vi "UTIL_Test_LUT.vi"() -> ()   [LabVIEW 2024]
uses:
  Control Definitions/Def FullCfg.ctl
  Control Definitions/Def BenchCfg.ctl
  Control Definitions/Def PumpCtlRefs.ctl
  Control Definitions/Def Bench Status.ctl
  Control Definitions/Ded Spec RNG.ctl
  Control Definitions/Ded LUT_Status.ctl
panel:
  out "Spec RNG":T1={"Specs"=[6.885, 6.785, 6.435, 304.0, 296.0], "Index(n)"=2, "LUT Status"={"ChA/!ChB"=FALSE, "Drain/!Fill"=FALSE, "In Range?"=TRUE, "Switch Range?"=FALSE, "Measure R?"=FALSE, "Vaild R?"=FALSE}, "Index(n-1)"=1}
  in  "Level IN inches":dbl=5.0
  in  "ChA/!ChB":bool
  in  "Drain!Fill":bool
  in  "Full Cfg":T3={"Bench Config"={"Name"="OLR001", {"Step Levels"=0.05, "Tolerance"=0.01, "Sample Rate"=0.05, "Resistor"=100.0, "M Level Cal"=1.0, "[B Level Cal"=0.0, "Max Fill Rate"=0.025, "Empty Inches"=8.6, "Full Inches"=2.0}}, "Test Value Table "=[[98.0, 102.0, 7.91, 8.01, 7.55, 7.65, 98.0, 102.0, 7.685, 7.785, 7.325, 7.425], [197.0, 203.0, 7.46, 7.56, 7.1, 7.2, 197.0, 203.0, 7.235, 7.335, 6.875, 6.975], [296.0, 304.0, 7.01, 7.11, 6.65, 6.75, 296.0, 304.0, 6.785, 6.885, 6.425, 6.525], [395.0, 405.0, 6.56, 6.66, 6.2, 6.3, 395.0, 405.0, 6.335, 6.435, 5.975, 6.075], [494.0, 506.0, 6.11, 6.21, 5.75, 5.85, 494.0, 506.0, 5.885, 5.985, 5.525, 5.625], [593.0, 607.0, 5.66, 5.76, 5.3, 5.4, 593.0, 607.0, 5.435, 5.535, 5.075, 5.175], [692.0, 708.0, 5.21, 5.31, 4.85, 4.95, 692.0, 708.0, 4.985, 5.085, 4.625, 4.725], [791.0, 809.0, 4.76, 4.86, 4.4, 4.5, 791.0, 809.0, 4.535, 4.635, 4.175, 4.275], [890.0, 910.0, 4.31, 4.41, 3.95, 4.05, 890.0, 910.0, 4.085, 4.185, 3.725, 3.825], [989.0, 1011.0, 3.86, 3.96, 3.5, 3.6, 989.0, 1011.0, 3.635, 3.735, 3.275, 3.375], [1088.0, 1112.0, 3.41, 3.51, 3.05, 3.15, 1088.0, 1112.0, 3.185, 3.285, 2.825, 2.925], [0.0, 0.0, 0.0, 0.0, 0.0, 0.0, 0.0, 0.0, 0.0, 0.0, 0.0, 0.0]], "Table Col Titles"=[["Aohm Lo", "Aohm Hi", "A Fill Lo", "A Fill Hi", "A Drain Lo", "A Drain Hi", "Bohm Lo", "Bohm Hi", "B Fill Lo", "B Fill Hi", "B Drain Lo", "B Drain Hi"]], "Pump CtlRef In"={"Fill "=refnum, "Drain"=refnum, "Level PV"=refnum, "Flow Rate%"=refnum, "Run Test"=refnum, "Sim"=refnum, "Jog"=refnum, "Level SP"=refnum}, "Bench Status"={"Pump Status"=refnum, "Instrumnet\n Status"=refnum}}
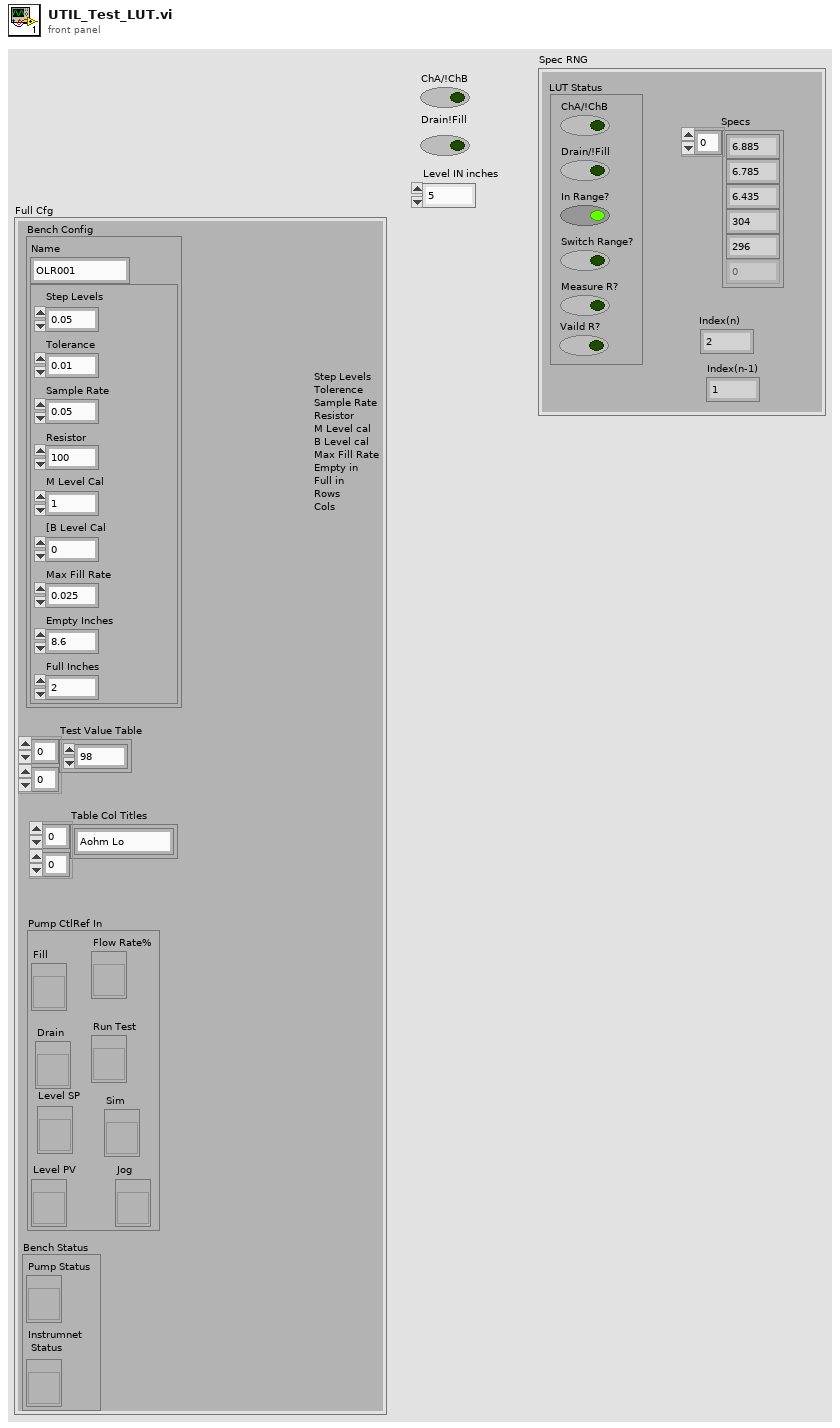
[diagram p1: front panel]
types:
  T1 = typedef "Ded Spec RNG.ctl" = cluster{"Specs":dbl[], "Index(n)":i32, "LUT Status":T2, "Index(n-1)":i32}
  T2 = typedef "Ded LUT_Status.ctl" = cluster{"ChA/!ChB":bool, "Drain/!Fill":bool, "In Range?":bool, "Switch Range?":bool, "Measure R?":bool, "Vaild R?":bool}
  T3 = typedef "Def FullCfg.ctl" = cluster{"Bench Config":T4, "Test Value Table ":dbl[][], "Table Col Titles":string[][], "Pump CtlRef In":T5, "Bench Status":T6}
  T4 = typedef "Def BenchCfg.ctl" = cluster{"Name":string, cluster{"Step Levels":dbl, "Tolerance":dbl, "Sample Rate":dbl, "Resistor":dbl, "M Level Cal":dbl, "[B Level Cal":dbl, "Max Fill Rate":dbl, "Empty Inches":dbl, "Full Inches":dbl}}
  T5 = typedef "Def PumpCtlRefs.ctl" = cluster{"Fill ":refnum<vi>, "Drain":refnum<vi>, "Level PV":refnum<vi>, "Flow Rate%":refnum<vi>, "Run Test":refnum<vi>, "Sim":refnum<vi>, "Jog":refnum<vi>, "Level SP":refnum<vi>}
  T6 = typedef "Def Bench Status.ctl" = cluster{"Pump Status":refnum<vi>, "Instrumnet\n Status":refnum<vi>}
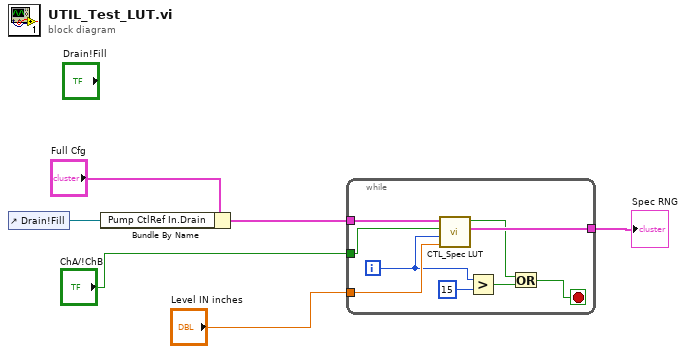
[diagram p0: block diagram]
diagram:
  n1 = control-ref of="Drain!Fill"() -> (w5:refnum<vi>)
  n2 = Bundle By Name(cluster="Full Cfg", "Pump CtlRef In.Drain"=w5) -> (w4:T3)
  n3 = while {
    tunnel: w4 -> [w15]
    tunnel: "ChA/!ChB" -> [w14]
    tunnel: "Level IN inches" -> [w13]
    tunnel: [w12] -> w1
    i -> [w11]
    stop <- w8 stop-if-true
    n4 = call "CTL_Spec LUT.vi"("Level IN inches"=w13, "Index"=w11, "ChA/!ChB"=w14, "Full Cfg"=w15) -> ("Spec RNG"=w12:T1, "In Range?"=w7:bool)  [unwired: 6 in]
    n5 = Greater?(x=w11, y=15) -> (0:w9:bool)
    n6 = Or(x=w7, y=w9) -> (x .or. y?=w8:bool)
  }
  "Spec RNG" <- w1
